vi "Acknowledge Completion.vi"(8 "error in (no error)":errorcluster, 10 "VI Refnum":refnum<vi>, 11 "Async Methods Actor in":refnum<class "Async Methods Actor.lvclass">) -> (0 "error out":errorcluster, 3 "Async Methods Actor out":refnum<class "Async Methods Actor.lvclass">)   [LabVIEW 2021, in "Async Methods Actor.lvlib" / "Async Methods Actor.lvclass"]
uses:
  Async Methods Actor.lvclass
  <vilib>/ActorFramework/Actor/Actor.lvclass
  Async Methods Actor Messages/Async Message/Async Message.lvclass
  Async Methods Actor.lvclass/Async Methods Actor.ctl
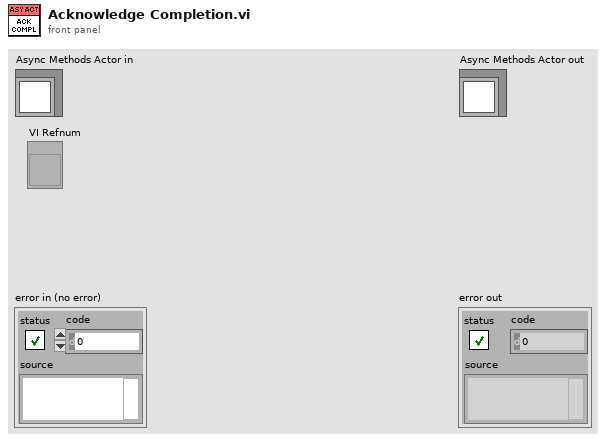
[diagram p1: front panel]
types:
  T1 = typedef "Async Methods Actor.lvlib/Async Methods Actor.lvclass/VI Refnums Map.ctl" = map{refnum<vi>, T2}
  T2 = typedef "Async Methods Actor.lvlib/Async Methods Actor.lvclass/VI Refnums Map Value.ctl" = cluster{"Async Call Method":T3, "VI Refnum Lifecycle":T4, "Message Path":path}
  T3 = typedef "Async Methods Actor.lvlib/Async Methods Actor.lvclass/Async Call Method.ctl" = enum16{"Call and Collect", "Call and Forget"}
  T4 = typedef "Async Methods Actor.lvlib/Async Methods Actor.lvclass/VI Refnum Lifecycle.ctl" = enum16{"Destroy on Exit", "Destroy on Actor Exit", "Leak"}
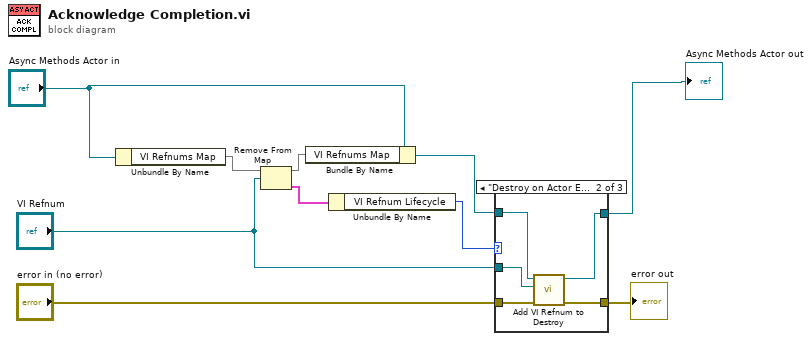
[diagram p0: block diagram]
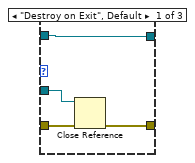
[diagram p2: hidden frame]
diagram:
  n1 = Unbundle By Name("Async Methods Actor in") -> ("VI Refnums Map"=w10:T1)
  n2 = Remove From Map(10:"VI Refnum", 11:w10) -> (1:w7:T2, 3:w9:T1)  [unwired: 1 out]
  n3 = Bundle By Name(cluster="Async Methods Actor in", "VI Refnums Map"=w9) -> (w2:refnum<class "Async Methods Actor.lvclass">)
  n4 = Unbundle By Name(w7) -> ("VI Refnum Lifecycle"=w6:T4)
  n5 = case shown="\"Destroy on Actor Exit\"" w6 {
    tunnel: "VI Refnum" -> [w14 w17 _]
    tunnel: "error in (no error)" -> [w13 w19 w20]
    tunnel: [w12 w18 w20] -> w3
    tunnel: w2 -> [w11 w16 w21]
    tunnel: [w11 w15 w21] -> w1
    frame "Destroy on Exit", Default {
      n6 = Close Reference(reference=w14, error in (no error)=w13) -> (error out=w12:errorcluster)
    }
    frame "Destroy on Actor Exit" {
      n7 = call "Add VI Refnum to Destroy.vi"("error in (no error)"=w19, "key type"=w17, "Async Methods Actor in"=w16) -> ("error out"=w18:errorcluster, "Async Methods Actor out"=w15:refnum<class "Async Methods Actor.lvclass">)  [unwired: 7 in]
    }
    frame "Leak" {
    }
  }
  "error out" <- w3
  "Async Methods Actor out" <- w1
